vi "SavePlotData.vi"(8 "error in (no error)":errorcluster caption="错误输入（无错误）", 10 "数据输入":waveform(dbl)[](array[waveform]), 11 "TPlot 输入":refnum<class "TPlot.lvclass">) -> (0 "error out":errorcluster caption="错误输出", 3 "TPlot 输出":refnum<class "TPlot.lvclass">)   [LabVIEW 2018, in "DataDisplay.lvlib" / "TPlot.lvclass"]
uses:
  TPlot.lvclass
  TPlot.lvclass/TPlot.ctl
  SubVI/WriteDataFile.vi
  DataDisplay.lvlib
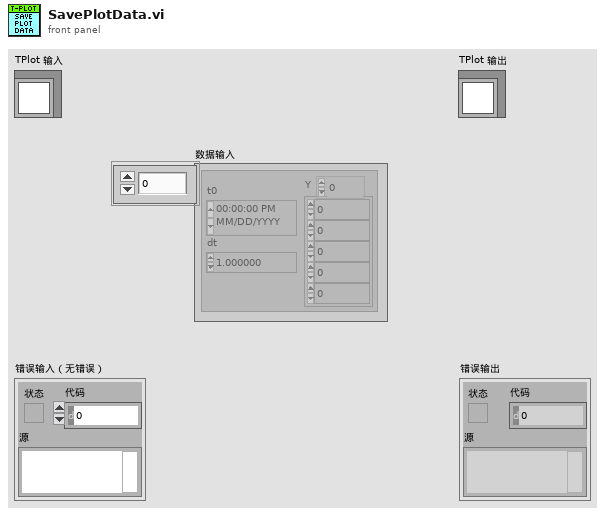
[diagram p1: front panel]
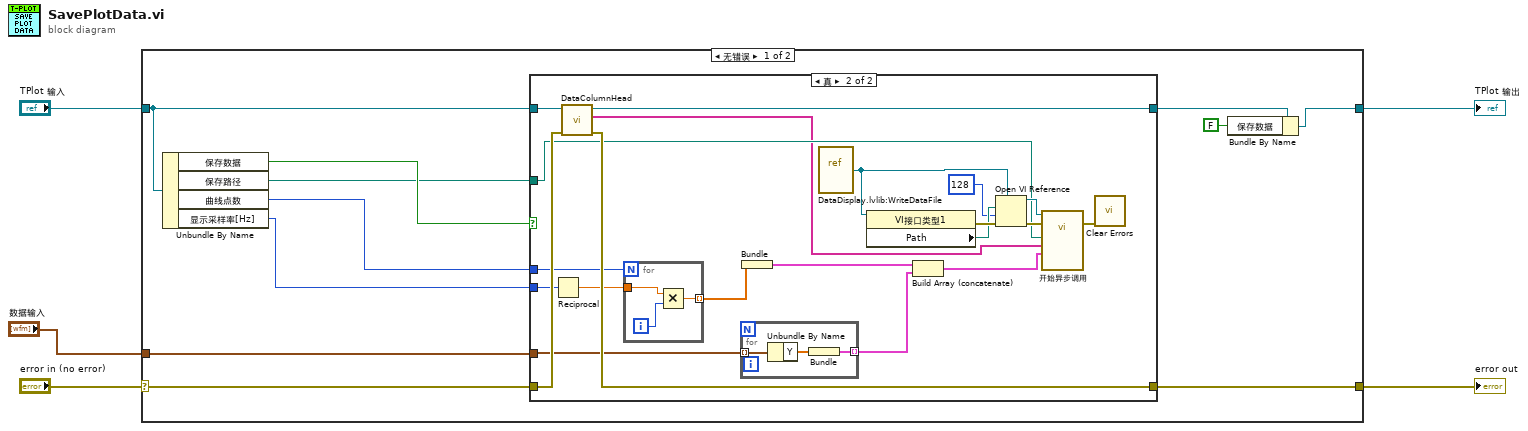
[diagram p0: block diagram]
diagram:
  n1 = case shown="无错误" "error in (no error)" {
    selector: "error in (no error)" -> [w10 w47]
    tunnel: [w9 w47] -> w4
    tunnel: [w11 w46] -> w2
    tunnel: "TPlot 输入" -> [w13 w46]
    tunnel: "数据输入" -> [w8 _]
    frame No Error {
      n2 = Unbundle By Name(w13) -> ("保存数据"=w16:bool, "保存路径"=w14:path, "曲线点数"=w6:i32, "显示采样率[Hz]"=w7:i32)
      n3 = case shown="真" w16 {
        tunnel: w14 -> [_ w29]
        tunnel: [w17 w38] -> w12
        tunnel: w13 -> [w17 w39]
        tunnel: [w18 w36] -> w9
        tunnel: w10 -> [w18 w37]
        tunnel: w8 -> [_ w19]
        tunnel: w7 -> [_ w23]
        tunnel: w6 -> [_ w22]
        frame False {
        }
        frame True {
          n4 = Reciprocal(x=w23) -> (1/x=w24:dbl)
          n5 = call "DataColumnHead.vi"("error in (no error)"=w37, "TPlot 输入"=w39) -> ("error out"=w36:errorcluster, "首行"=w28:string[], "TPlot 输出"=w38:refnum<class "TPlot.lvclass">)  [unwired: 7 in]
          n6 = for {
            N: w22 -> [_]
            tunnel: w24 -> [w44]
            tunnel: [w43] -> w25 mode=indexing
            i -> [w45]
            n7 = Multiply(x=w44, y=w45) -> (x*y=w43:dbl)
          }
          n8 = for {
            tunnel: w19 -> [w42] mode=indexing
            tunnel: [w40] -> w20 mode=indexing
            n9 = Unbundle By Name(w42) -> ("Y"=w41:dbl[])
            n10 = Bundle("Y"=w41) -> (w40:cluster{"Y":dbl[]})  [unwired: 1 in]
          }
          n11 = Bundle(w25) -> (w21:cluster{dbl[]})  [unwired: 1 in]
          n12 = vi-ref "DataDisplay.lvlib:WriteDataFile.vi"() -> (w34:refnum<vi>)
          n13 = property class="VI接口类型1"(reference=w34) -> (error out=w35:errorcluster, "Path"=w33:path)  [unwired: 1 in, 1 out]
          n14 = Build Array (concatenate)(w21, w20) -> (w26:cluster{"Y":dbl[]}[])
          n15 = Open VI Reference(type specifier VI Refnum (for type only)=w34, vi path=w33, options=128 ("选项"), error in (no error)=w35) -> (vi reference=w31:refnum<vi>, error out=w30:errorcluster)  [unwired: 2 in]
          n16 = call-by-ref "开始异步调用"(reference=w31, error in=w30, "数据输入"=w26, "首行"=w28, "保存路径"=w29) -> (error out=w27:errorcluster)  [unwired: 9 in, 1 out]
          n17 = call <vilib>:"Clear Errors.vi"("error in (no error)"=w27) -> ()  [unwired: 5 in, 2 out]
        }
      }
      n18 = Bundle By Name(cluster=w12, "保存数据"=FALSE) -> (w11:refnum<class "TPlot.lvclass">)
    }
    frame Error {
    }
  }
  "error out" <- w4
  "TPlot 输出" <- w2
